vi "CLSUIP_GetIndexArrayNodes.vi"(8 "error in (no error)":errorcluster, 11 "VI Refnum":refnum<vi>) -> (0 "error out":errorcluster, 2 "IndexArray Refs":refnum<vi>[](array[refnum]), 3 "VI Refnum out":refnum<vi>)   [LabVIEW 2021, in "MemberVICreation.lvlib"]
uses:
  <resource>/Framework/Providers/LVClassLibrary/NewAccessors/MemberVICreation.lvlib
  <vilib>/Utility/traverseref.llb/TRef TravTarget.ctl
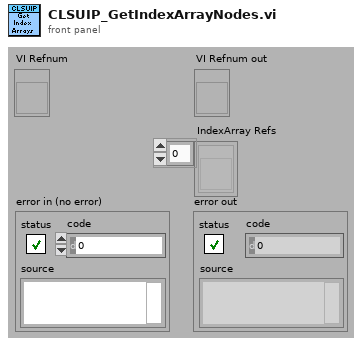
[diagram p1: front panel]
types:
  T1 = typedef "TRef TravTarget.ctl" = enum16{"FP", "BD", "Other"}
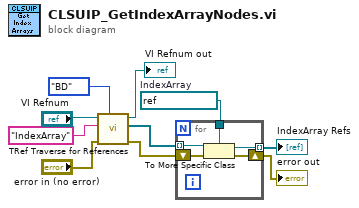
[diagram p0: block diagram]
diagram:
  w4 = refnum<vi> refnum  # IndexArray
  n1 = call <vilib>:"TRef Traverse for References.vi"("Traverse Target"=TRef_TravTarget."BD", "error in (no error)"="error in (no error)", "Class Name"="IndexArray" ("y"), "VI Refnum"="VI Refnum") -> ("error out"=w5:errorcluster, "References"=w6:refnum<vi>[], "dup VI Refnum"=→"VI Refnum out":refnum<vi>)  [unwired: 1 in, 4 out]
  n2 = for {
    tunnel: w6 -> [w15] mode=indexing
    shift-right: [w13] -> w2
    shift-left: w5 -> [w14]
    tunnel: w4 -> [w12]
    tunnel: [w11] -> w3 mode=indexing
    n3 = To More Specific Class(target class=w12, reference=w15, error in=w14) -> (specific class reference=w11:refnum<vi>, error out=w13:errorcluster)
  }
  "error out" <- w2
  "IndexArray Refs" <- w3
